vi "Core Usage.vi"(11 "Error In":errorcluster {"Code" format="%.0x"}) -> (15 "Error Out":errorcluster {"Code" format="%.0x"})   [LabVIEW 2020, in "Core.lvlib" / "Core.lvclass"]
doc: "Sample usage of this class."
uses:
  Core.lvclass
panel:
  # "/* General */"
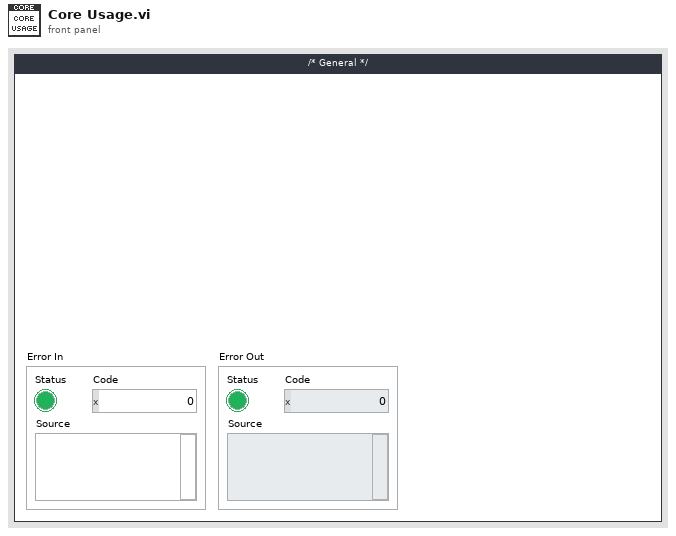
[diagram p1: front panel]
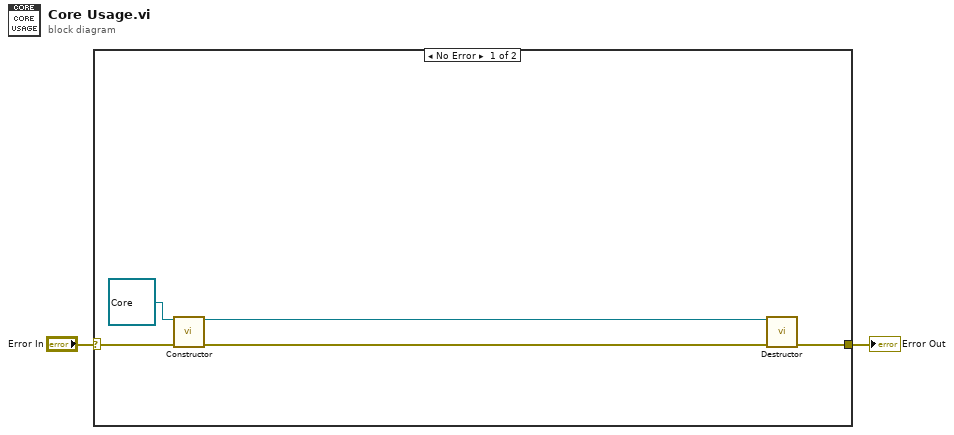
[diagram p0: block diagram]
diagram:
  n1 = case shown="No Error" "Error In" {
    selector: "Error In" -> [w6 w8]
    tunnel: [w7 w8] -> w1
    frame No Error {
      n2 = call-dynamic "Constructor.vi"("Core In"=refnum<class "Core.lvclass"> refnum ("Core.lvlib:Core"), "Error In"=w6) -> ("Core Out"=w4:refnum<class "Core.lvclass">, "Error Out"=w5:errorcluster)  [unwired: 12 in]
      n3 = call-dynamic "Destructor.vi"("Core In"=w4, "Error In"=w5) -> ("Error Out"=w7:errorcluster)  [unwired: 12 in, 1 out]
    }
    frame Error {
    }
  }
  "Error Out" <- w1
